vi "FPGA Open Reference By TypeDef.vi"(6 "max num IRQs":i32=1, 7 "Run?":T1, 8 "error in (no error)":errorcluster, 10 "FPGA Resource":string="RIO0", 11 "Bitfile Path":path) -> (0 "error out":errorcluster, 3 "FPGA Session":refnum<class "FPGA Interface By TypeDefs.lvclass">)   [LabVIEW 2010, in "FPGA Interface By TypeDefs.lvclass"]
uses:
  FPGA Interface By TypeDefs.lvclass
  <userlib>/_FPGA Interface Advanced Tools/FPGA Interface Wrapper/TypeDefs/Open Attribute.ctl
  <userlib>/_FPGA Interface Advanced Tools/FPGA Interface Base/TypeDefs/FPGA Register Names.ctl
  <userlib>/_FPGA Interface Advanced Tools/FPGA Interface Base/FPGA Interface Base.lvclass
  <userlib>/_FPGA Interface Advanced Tools/FPGA Interface Wrapper/FPGA Interface Wrapper.lvlib
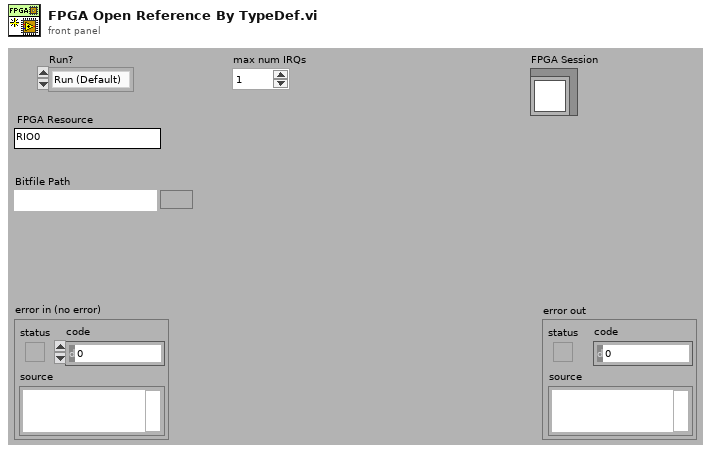
[diagram p1: front panel]
types:
  T1 = typedef "FPGA Interface Wrapper.lvlib/Open Attribute.ctl" = enum32{"Run (Default)", "No Run"}
  T2 = typedef "FPGA Interface Base.lvclass/FPGA Register Names.ctl" = cluster{"Indicators":string[], "Controls":string[], "TargetToHost FIFOs":string[], "HostToTarget FIFOs":string[]}
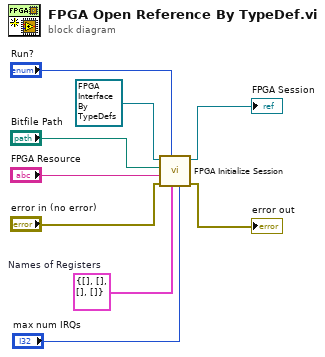
[diagram p0: block diagram]
diagram:
  w6 = T2 {"Indicators"=[], "Controls"=[], "TargetToHost FIFOs"=[], "HostToTarget FIFOs"=[]}  # Names of Registers
  n1 = call-dynamic "FPGA Initialize Session.vi"("max num IRQs"="max num IRQs", "Names of Registers"=w6, "Run?"="Run?", "error in (no error)"="error in (no error)", "FPGA Resource"="FPGA Resource", "Bitfile Path"="Bitfile Path", "FPGA Interface Base In"=refnum<class "FPGA Interface By TypeDefs.lvclass"> refnum ("FPGA Interface By TypeDefs.lvclass")) -> ("error out"=→"error out":errorcluster, "FPGA Interface Base Out"=→"FPGA Session":refnum<class "FPGA Interface By TypeDefs.lvclass">)  [unwired: 3 in]
